vi "parse_dep_vars.vi"(8 "error in (no error)":errorcluster, 11 "ExperimentVariables in":refnum<class "ExperimentVariables.lvclass">) -> (0 "error out":errorcluster, 2 "Variable Settings (out)":T1={"Measurements per Iteration"=1, "Local Data Path"=path "C:/Users/Saffmanlab/Documents/Cesium/data", "Experiment description suffix for filename (no spaces please)"="", "Network Data Path"=path "Z:/", "Copy data to network"=TRUE, "Measurement Timeout (ms)"=0, "Independent Variables"=[], "Dependent Variables"=[], "Run Test Mode"=FALSE} {"Independent Variables"."# steps" min=1 step=1; "Measurements per Iteration" min=1 step=1}, 3 "ExperimentVariables out":refnum<class "ExperimentVariables.lvclass">)   [LabVIEW 2013]
uses:
  ExperimentVariables.lvclass
  Variable_Settings.ctl
panel:
  # "Parameters will be evaluated once at the beginning of the experiment from top to bottom, \nso any parameter may depend on all those above it.\nVariables will be evaluated each iteration.\nParameters and Variables may be used in various other experiment settings, as noted.\nSee LabView Help -> Formula Node and Expression Node Functions for a list of available functions."
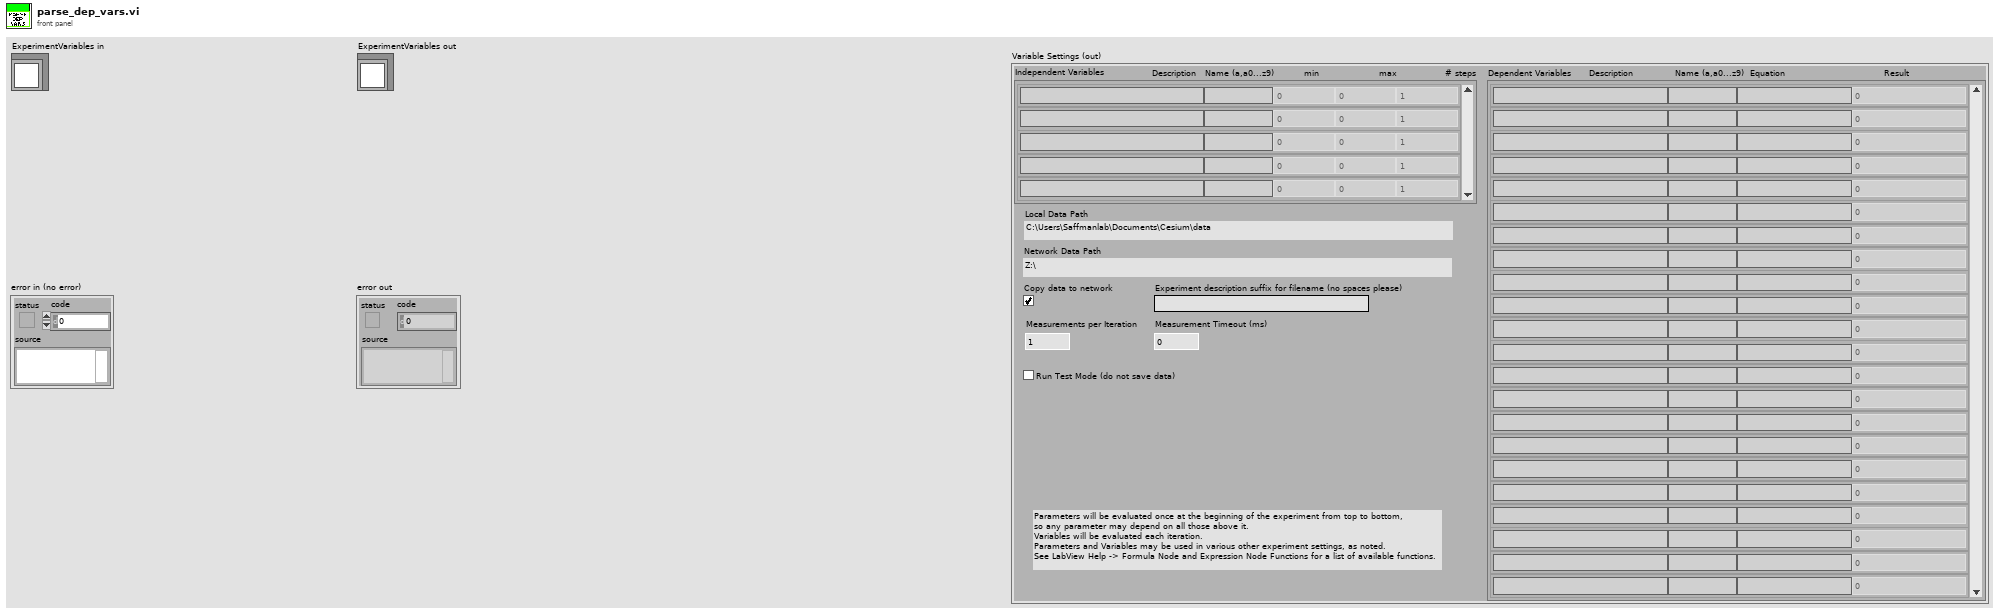
[diagram p1: front panel]
types:
  T1 = typedef "ExperimentVariables.lvclass/Variable_Settings.ctl" = cluster{"Measurements per Iteration":i32, "Local Data Path":path, "Experiment description suffix for filename (no spaces please)":string, "Network Data Path":path, "Copy data to network":bool, "Measurement Timeout (ms)":u32, "Independent Variables":cluster{"Description":string, "Name (a,a0...a9)":string, "min":dbl, "max":dbl, "# steps":u32}[], "Dependent Variables":cluster{"Description":string, "Name (a,a0...a9)":string, "Equation":string, "Result":dbl}[], "Run Test Mode":bool}
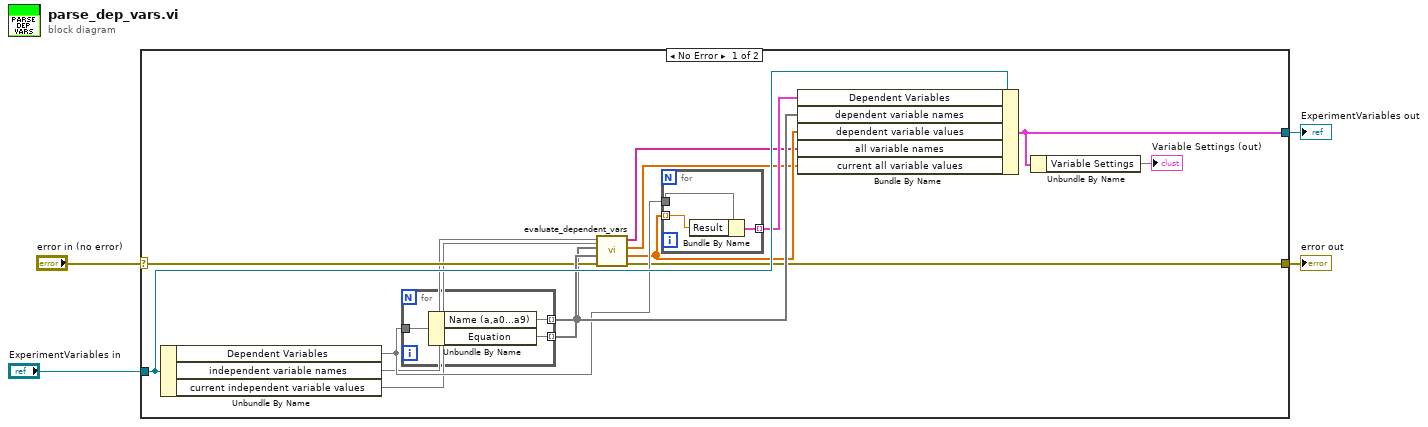
[diagram p0: block diagram]
diagram:
  n1 = case shown="No Error" "error in (no error)" {
    selector: "error in (no error)" -> [w16 w26]
    tunnel: [w10 w26] -> w3
    tunnel: [w13 w25] -> w1
    tunnel: "ExperimentVariables in" -> [w18 w25]
    frame No Error {
      n2 = Unbundle By Name(w18) -> ("Dependent Variables"=w14, "independent variable names"=w9, "current independent variable values"=w8)
      n3 = for {
        tunnel: w14 -> [w24]
        tunnel: [w23] -> w15 mode=indexing
        tunnel: [w22] -> w17 mode=indexing
        n4 = Unbundle By Name(w24) -> ("Name (a,a0...a9)"=w23, "Equation"=w22)
      }
      n5 = call "evaluate_dependent_vars.vi"("current independent variable values"=w8, "error in (no error)"=w16, "dependent variable equations"=w17, "dependent variable names"=w15, "independent variable names"=w9) -> ("error out"=w10:errorcluster, "dependent variable results"=w7:dbl[], "current all variable values"=w6:dbl[], "all variable names"=w5:string[])  [unwired: 3 in]
      n6 = for {
        tunnel: w14 -> [w21]
        tunnel: w7 -> [w20] mode=indexing
        tunnel: [w19] -> w11 mode=indexing
        n7 = Bundle By Name(cluster=w21, "Result"=w20) -> (w19:cluster{})
      }
      n8 = Bundle By Name(cluster=w18, "Dependent Variables"=w11, "dependent variable names"=w15, "dependent variable values"=w7, "all variable names"=w5, "current all variable values"=w6) -> (w13:cluster{})
      n9 = Unbundle By Name(w13) -> ("Variable Settings"=→"Variable Settings (out)")
    }
    frame Error {
    }
  }
  "error out" <- w3
  "ExperimentVariables out" <- w1
